vi "Scan all.vi"(8 "error in (no error)":errorcluster, 10 "Start/Stop":bool, 11 "VISA resource name":refnum<visa-resource-name>) -> (0 "error out":errorcluster, 3 "VISA resource name out":refnum<visa-resource-name>)   [LabVIEW 2013, in "Fluke 2625A.lvlib"]
uses:
  <instrlib>/Fluke 2625A/Fluke 2625A.lvlib
panel:
  out "concatenated string":string
  out "Read Buffer total":string[](array[string])
  out "read buffer":string
  out "number":i32
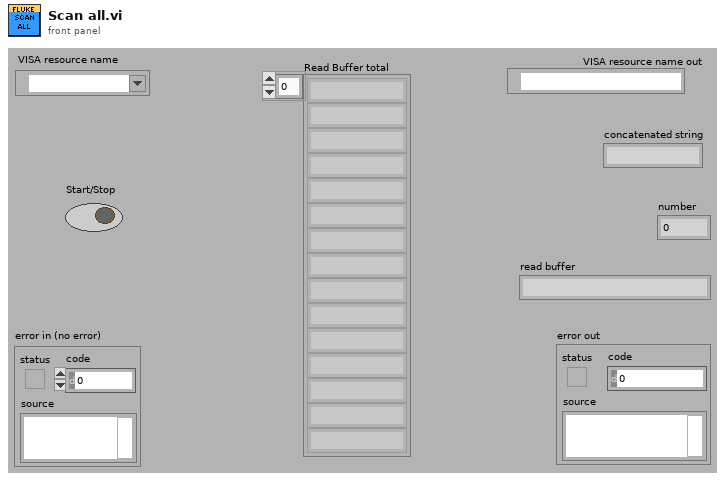
[diagram p1: front panel]
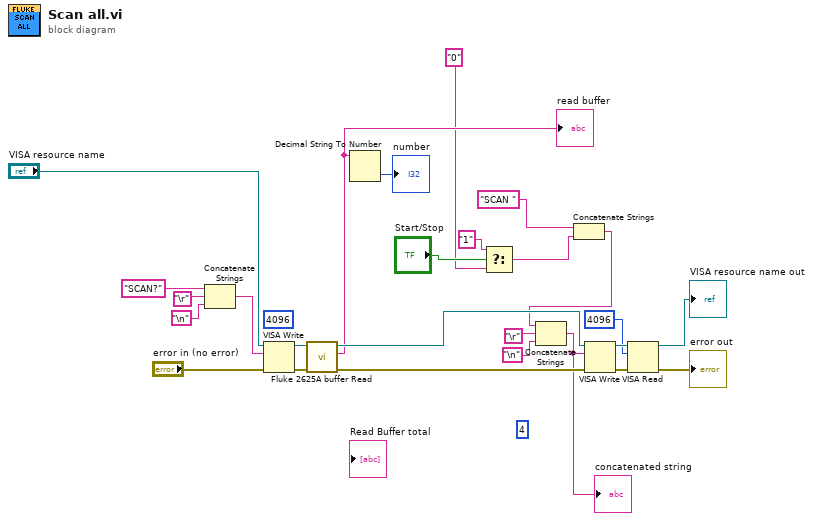
[diagram p0: block diagram]
diagram:
  (unwired) u32 4096 ("byte count")
  (unwired) u32 4 ("byte count")
  n1 = Concatenate Strings("SCAN?" ("write buffer"), "\r", "\n") -> (w25:string)
  n2 = VISA Write(VISA resource name="VISA resource name", write buffer=w25, error in (no error)="error in (no error)") -> (VISA resource name out=w17:refnum<visa-resource-name>, error out=w16:errorcluster)  [unwired: 1 out]
  n3 = call <instrlib>:"Fluke 2625A buffer Read.vi"("error out"=w16, "VISA resource name out"=w17) -> ("error out 2"=w14:errorcluster, "read buffer"=w13:string, "VISA resource name out 2"=w15:refnum<visa-resource-name>)  [unwired: 7 in]
  "read buffer" <- w13
  n4 = Decimal String To Number(string=w13) -> (number=→"number":i32)  [unwired: 2 in, 1 out]
  n5 = Select(t="1" ("write buffer"), s="Start/Stop", f="0" ("write buffer")) -> (s? t:f=w2:string)
  n6 = Concatenate Strings("SCAN " ("write buffer"), w2) -> (w1:string)
  n7 = Concatenate Strings(w1, "\r", "\n") -> (w11:string)
  "concatenated string" <- w11
  n8 = VISA Write(VISA resource name=w15, write buffer=w11, error in (no error)=w14) -> (VISA resource name out=w9:refnum<visa-resource-name>, error out=w8:errorcluster)  [unwired: 1 out]
  n9 = VISA Read(VISA resource name=w9, byte count=u32 4096, error in (no error)=w8) -> (VISA resource name out=→"VISA resource name out":refnum<visa-resource-name>, error out=→"error out":errorcluster)  [unwired: 2 out]
